vi "Multi-Function-Ctr Retrigg Pulse Train Generation for AI Sample Clock.vi"() -> ()   [LabVIEW 2015]
doc: "I. Description:\nThis example demonstrates how to generate a finite retriggerable digital pulse train from a Counter to be used as the clock for Analog Input. This example utilizes two counters.\n\nII. Instructions for Running:\n1. Select the physical channel to correspond to where your signal is input on the DAQ device.\n2. Enter the minimum and maximum signal ranges.\nNote: For better accuracy, try to match the input range to the expected voltage level of the measured signal.\n3. Select the Counter Channel which corresponds to the counter you want to generate your AI clock from.\n4. Select the Source of the Clock for the acquisition as the output of the counter you chose in step 3.\n5. Set the Rate at which the counter will generate.\nNote: The Rate should be at least twice as fast as the maximum frequency component of the signal being acquired.\n6. Enter the number of Samples per Channel to acquire. This will also be the number of pulses generated by the counter.\n7. Select the Source of the Digital Start Trigger for the acquisition.\n8. Select the edge, rising or falling, on which to trigger.\n\nIII. Block Diagram Steps:\n1. Create an analog input voltage channel. Also, create a Counter Output channel to produce a Pulse in terms of Frequency. If the Idle State of the pulse is set to low the first transition of the generated signal is from low to high.\n2. Define the parameters for an External Clock Source. Additionally, define the sample mode to be continuous. Also, use the DAQmx Timing VI (Implicit) to configure the duration of the pulse generation and the number of pulses to generate.\n3. Use the DAQmx Trigger VI to configure a counter trigger to start on a digital edge.\n4. Configure a buffer which is 1000 plus the number of samples per channel. This is necessary when simulating retriggerable finite transfers with a continuous acquisition because DMA needs a slightly larger buffer than the Samples per Channel. \n5. Use a DAQmx Trigger Property Node to set the operation for retriggerable.\n6. Call the Start VI to begin the acquisition and to arm the counter which begins the pulse train generation.\n7. Use the DAQ Read property node --> AvailSampPerChan to see how many samples have been acquired. If 'Samples per Channel' number of samples have been acquired, as you can set on the front panel, then Read the data, otherwise continue looping. This allows the user to stop the program by pressing the 'STOP' button at any time. \n8. Read the waveform data in a loop until the user hits the stop button or an error occurs.\nNote: This example reads data from one or more channels and returns an array of data. Use the Index Array function to access an individual channel of data.\n9. Call the Clear Task VI to clear the counter Task.\n10. Call the Clear Task VI to clear the AI Task.\n11. Use the popup dialog box to display an error if any.\n\nIV. I/O Connections Overview:\nMake sure your signal input terminal matches the Physical Channel I/O control. Note that there is no external wiring necessary to connect the counter output to the AI clock input. For further connection information, refer to your hardware reference manual."
uses:
  <vilib>/Utility/error.llb/DialogType.ctl
  <vilib>/DAQmx/read.llb/DAQmx Read (Analog 1D DBL 1Chan NSamp).vi
  <vilib>/DAQmx/create/channels.llb/DAQmx Create Channel (AI-Voltage-Basic).vi
  <vilib>/DAQmx/configure/timing.llb/DAQmx Timing (Sample Clock).vi
  <vilib>/DAQmx/create/channels.llb/DAQmx Create Channel (CO-Pulse Generation-Ticks).vi
  <vilib>/DAQmx/configure/timing.llb/DAQmx Timing (Implicit).vi
  <vilib>/DAQmx/configure/trigger.llb/DAQmx Start Trigger (Digital Edge).vi
  <vilib>/DAQmx/miscellaneous.llb/DAQmx Fill In Error Info.vi
  <resource>/objmgr/daqmx.rc
panel:
  out "Waveform Graph":dbl[](graph)
  in  "Stop":bool caption="stop"
  in  "Clock Source":tag="OnboardClock" caption="source"
  in  "Physical Channel":tag="PXI1Slot2/ai0"
  in  "Source":tag="/PXI1Slot2/ai/SampleClock" caption="Trigger Source"
  in  "Rate (Hz)":dbl=10000.0 format="%0.2f"
  in  "Counter Channel":tag="PXI1Slot2/ctr0"
  in  "Samples per Channel":u32=1000
  # "For instructions, select Help>>Show Context Help"
  # "Channel Parameters"
  # "Timing Parameters"
  # "Trigger Parameters"
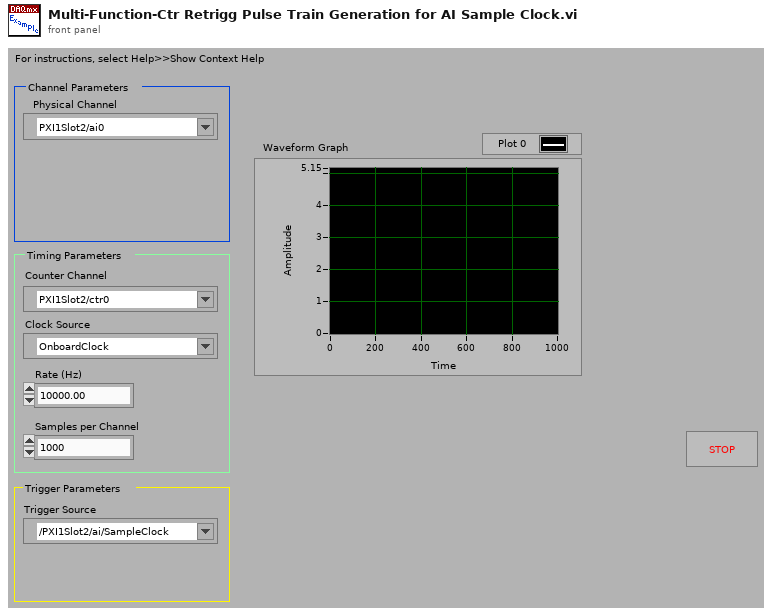
[diagram p1: front panel]
types:
  T1 = typedef "DialogType.ctl" = u16
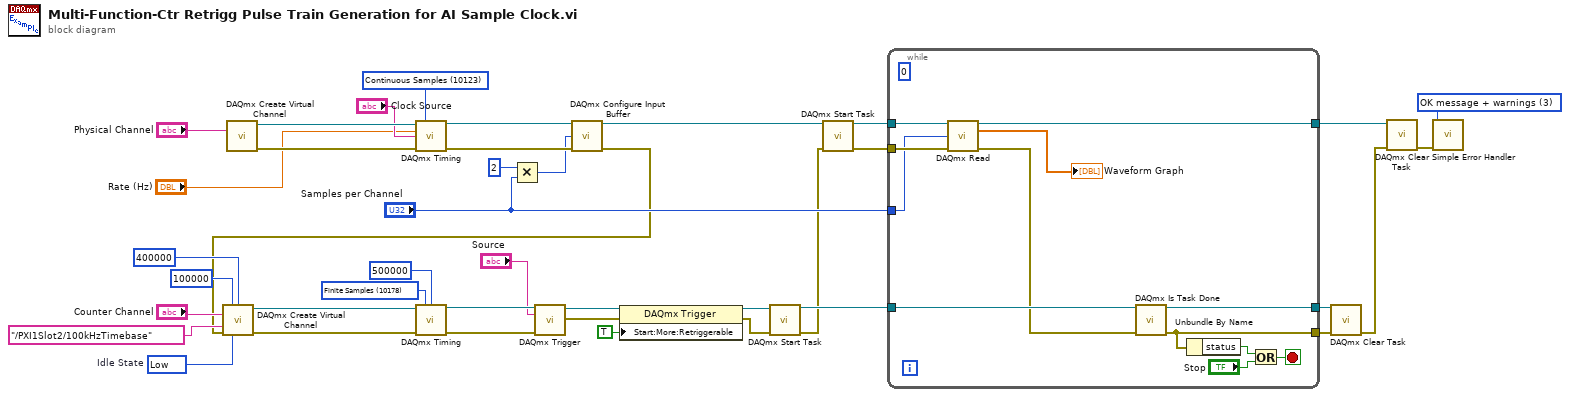
[diagram p0: block diagram]
diagram:
  w16 = T1 3 items=["no dialog", "OK message", "continue or stop message", "OK message + warnings", "continue/stop + warnings"] ("type of dialog (OK msg:1)")
  w36 = 10214 items=["High"=10192, "Low"=10214]  # Idle State
  w24 = 10123 items=["Finite Samples"=10178, "Continuous Samples"=10123] ("sample mode")
  w38 = 10178 items=["Finite Samples"=10178, "Continuous Samples"=10123] ("sample mode")
  n1 = call-poly <vilib>:"DAQmx Create Virtual Channel.vi"("physical channels"="Physical Channel") -> ("task out"=w26:refnum<k21>, "error out"=w27:errorcluster)  [unwired: 13 in]
  n2 = call-poly <vilib>:"DAQmx Timing.vi"("task/channels in"=w26, "sample mode"=w24, "rate"="Rate (Hz)", "source"="Clock Source", "error in"=w27) -> ("task out"=w15:refnum<k21>, "error out"=w14:errorcluster)  [unwired: 9 in]
  n3 = Multiply(x=u32 2, y="Samples per Channel") -> (x*y=w6:u32)
  n4 = call <vilib>:"DAQmx Configure Input Buffer.vi"("task/channels in"=w15, "buffer size (in samples per channel)"=w6, "error in"=w14) -> ("task out"=w12:refnum<k21>, "error out"=w3:errorcluster)  [unwired: 11 in]
  n5 = call-poly <vilib>:"DAQmx Create Virtual Channel.vi"("high ticks"=u32 100000, "low ticks"=u32 400000, "counter"="Counter Channel", "source of ticks"=tag "/PXI1Slot2/100kHzTimebase", "error in"=w3, "idle state"=w36) -> ("task out"=w39:refnum<k21>, "error out"=w40:errorcluster)  [unwired: 8 in]
  n6 = call-poly <vilib>:"DAQmx Timing.vi"("task/channels in"=w39, "sample mode"=w38, "samples per channel"=500000, "error in"=w40) -> ("task out"=w35:refnum<k21>, "error out"=w34:errorcluster)  [unwired: 10 in]
  n7 = call-poly <vilib>:"DAQmx Trigger.vi"("task/channels in"=w35, "source"="Source", "error in"=w34) -> ("task out"=w31:refnum<k21>, "error out"=w30:errorcluster)  [unwired: 11 in]
  n8 = property class="DAQmx Trigger"(reference=w31, error in=w30, "Start:More:Retriggerable"=TRUE) -> (reference out=w29:refnum<k21>, error out=w28:errorcluster)
  n9 = call <vilib>:"DAQmx Start Task.vi"("task/channels in"=w29, "error in"=w28) -> ("task out"=w21:refnum<k21>, "error out"=w2:errorcluster)  [unwired: 12 in]
  n10 = call <vilib>:"DAQmx Start Task.vi"("task/channels in"=w12, "error in"=w2) -> ("task out"=w13:refnum<k21>, "error out"=w1:errorcluster)  [unwired: 12 in]
  n11 = while {
    tunnel: w13 -> [w46]
    tunnel: w1 -> [w45]
    tunnel: [w47] -> w20
    tunnel: w21 -> [w49]
    tunnel: [w48] -> w19
    tunnel: [w44] -> w8
    tunnel: "Samples per Channel" -> [w42]
    stop <- w51 stop-if-true
    (unwired) 0
    n12 = call-poly <vilib>:"DAQmx Read.vi"("task/channels in"=w46, "number of samples per channel"=w42, "error in"=w45) -> ("task out"=w44:refnum<k21>, "data"=→"Waveform Graph":dbl[], "error out"=w43:errorcluster)  [unwired: 10 in]
    n13 = call <vilib>:"DAQmx Is Task Done.vi"("task/channels in"=w49, "error in"=w43) -> ("task out"=w47:refnum<k21>, "error out"=w48:errorcluster)  [unwired: 11 in, 1 out]
    n14 = Unbundle By Name(w48) -> ("status"=w50:bool)
    n15 = Or(x=w50, y="Stop") -> (x .or. y?=w51:bool)
  }
  n16 = call <vilib>:"DAQmx Clear Task.vi"("task in"=w20, "error in"=w19) -> ("error out"=w18:errorcluster)  [unwired: 13 in]
  n17 = call <vilib>:"DAQmx Clear Task.vi"("task in"=w8, "error in"=w18) -> ("error out"=w17:errorcluster)  [unwired: 13 in]
  n18 = call <vilib>:"Simple Error Handler.vi"("type of dialog (OK msg:1)"=w16, "error in (no error)"=w17) -> ()  [unwired: 3 in, 5 out]
